vi "Window Properties.vi"   [LabVIEW 2010, in "NI_AALPro.lvlib"]
doc: "Computes the coherent gain and equivalent noise bandwidth of a window. You must manually select the polymorphic instance you want to use."
uses:
  NI_AALPro.lvlib
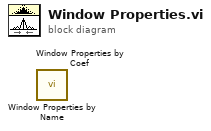
[diagram p0: block diagram]
diagram:
  n1 = call "Window Properties by Name.vi"() -> ()  [unwired: 9 in, 3 out]
  n2 = call "Window Properties by Coef.vi"() -> ()  [unwired: 9 in, 3 out]
